vi "mail_number_upload_system_dev.vi"() -> ()   [LabVIEW 2011]
doc: "This example opens a connection to a database specified by the Connection string (replace the DNS name with your database) inserts a new row into the table \"myOtherTable\" (replace the SQL string with your own SQL query)."
panel:
  out "上傳結果：":string
  in  "輸入郵件編號":string
  out "錯誤訊息":cluster{"狀態":bool, "錯誤訊息碼":i32, "錯誤內容":string}
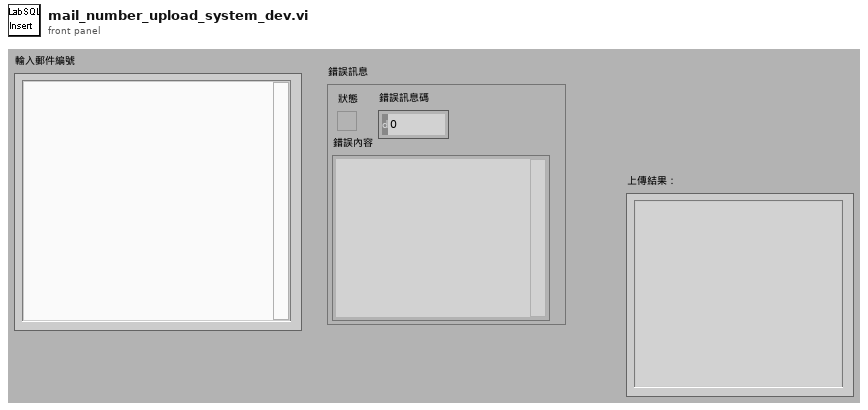
[diagram p1: front panel]
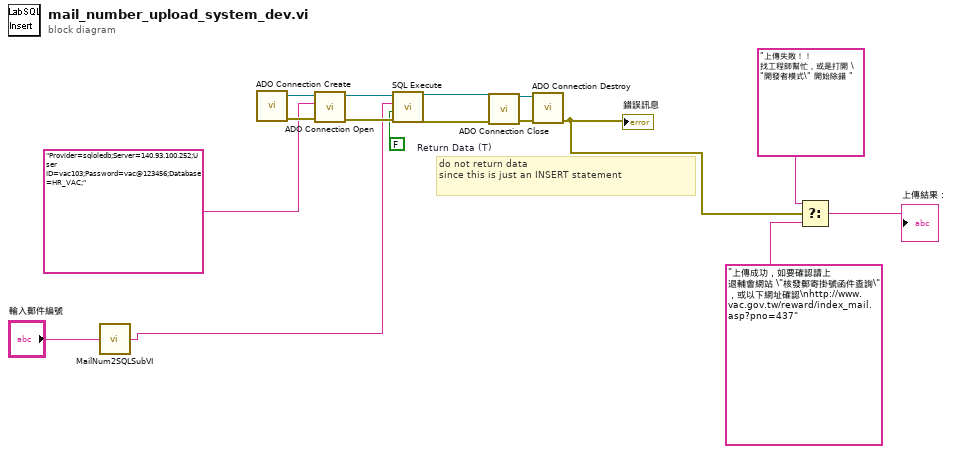
[diagram p0: block diagram]
diagram:
  w8 = FALSE  # Return Data (T)
  # "do not return data\nsince this is just an INSERT statement"
  n1 = call "MailNum2SQLSubVI.vi"("mail numbers"="輸入郵件編號") -> ("String"=w5:string)
  n2 = call "ADO Connection Create.vi"() -> ("error out"=w15:errorcluster, "ADODB._Connection Out"=w16:refnum<k7>)  [unwired: 10 in]
  n3 = call "ADO Connection Open.vi"("error in (no error)"=w15, "ConnectionString"="Provider=sqloledb;Server=140.93.100.252;User ID=vac103;Password=vac@123456;Database=HR_VAC;" ("ConnectionString 2"), "ADODB._Connection In"=w16) -> ("error out"=w13:errorcluster, "ADODB._Connection Out"=w14:refnum<k7>)  [unwired: 7 in]
  n4 = call "SQL Execute.vi"("error in (no error)"=w13, "Return Data (T)"=w8, "Command Text"=w5, "ADODB._Connection In"=w14) -> ("error out"=w12:errorcluster, "ADODB._Connection Out"=w11:refnum<k7>)  [unwired: 4 in, 2 out]
  n5 = call "ADO Connection Close.vi"("error in (no error)"=w12, "ADODB._Connection In"=w11) -> ("error out"=w10:errorcluster, "ADODB._Connection Out"=w9:refnum<k7>)  [unwired: 8 in]
  n6 = call "ADO Connection Destroy.vi"("error in (no error)"=w10, "ADODB._Connection In"=w9) -> ("error out"=w1:errorcluster)  [unwired: 9 in]
  "錯誤訊息" <- w1
  n7 = Select(t="上傳失敗！！ 找工程師幫忙，或是打開 \"開發者模式\" 開始除錯 " ("f"), s=w1, f="上傳成功，如要確認請上 退輔會網站 \"核發郵寄掛號函件查詢\" ，或以下網址確認\nhttp://www.vac.gov.tw/reward/index_mail.asp?pno=437" ("上傳結果：")) -> (s? t:f=→"上傳結果：":string)
